vi "USB3 Stop Acquisition.vi"(8 "error in (no error)":errorcluster, 11 "hCamera":u64) -> (0 "error out":errorcluster, 2 "function return":i32, 3 "hCamera out":u64)   [LabVIEW 2013, in "Octoplus_LIDAR.lvlib"]
doc: "CAMCMOSOCTUSB3_API int __cdecl USB3_StopAcquisition(CAM_HANDLE hCamera);"
uses:
  <userlib>/Octoplus_LIDAR/Octoplus_LIDAR.lvlib
  <userlib>/Octoplus_LIDAR/CamCmosOctUsb3.dll
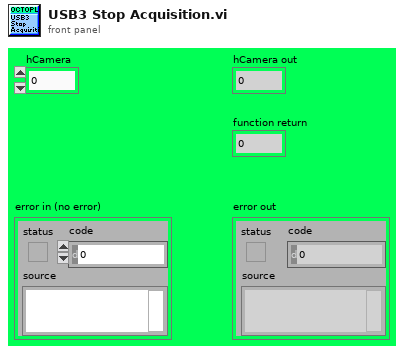
[diagram p1: front panel]
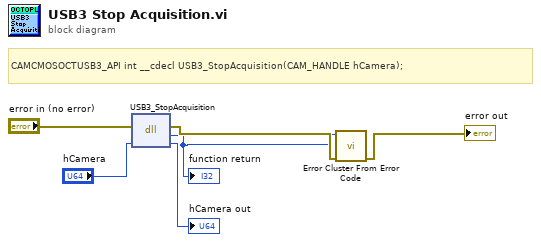
[diagram p0: block diagram]
diagram:
  # "CAMCMOSOCTUSB3_API int __cdecl USB3_StopAcquisition(CAM_HANDLE hCamera);"
  n1 = dll-call lib="C:/Program Files/National Instruments/LabVIEW 2013/user.lib/Octoplus_LIDAR/CamCmosOctUsb3.*" fn="USB3_StopAcquisition"(error in="error in (no error)", "hCamera"="hCamera") -> (error out=w3:errorcluster, "return type"=w1:i32, "hCamera"=→"hCamera out":u64)  [unwired: 2 in, 1 out]
  "function return" <- w1
  n2 = call <vilib>:"Error Cluster From Error Code.vi"("error in (no error)"=w3, "error code (0)"=w1) -> ("error out"=→"error out":errorcluster)  [unwired: 7 in]
